vi "Open Protocol.vi"(8 "error in (no error)":errorcluster, 11 "Python Protocol in":refnum<class "Python Protocol.lvclass">) -> (0 "error out":errorcluster, 3 "Python Protocol out":refnum<class "Python Protocol.lvclass">)   [LabVIEW 2012, in "Python Protocol Actor.lvlib" / "Python Protocol.lvclass"]
uses:
  Python Protocol.lvclass
  Python Protocol.lvclass/Python Protocol.ctl
  Read Compiler.vi
  Read Code.vi
  Read Path.vi
  Read Open.vi
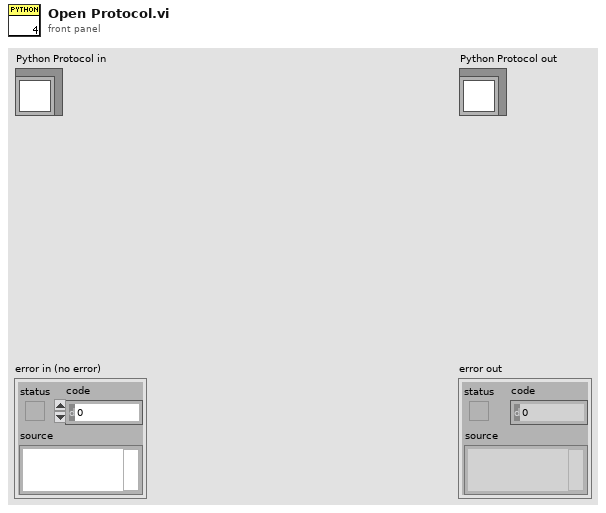
[diagram p1: front panel]
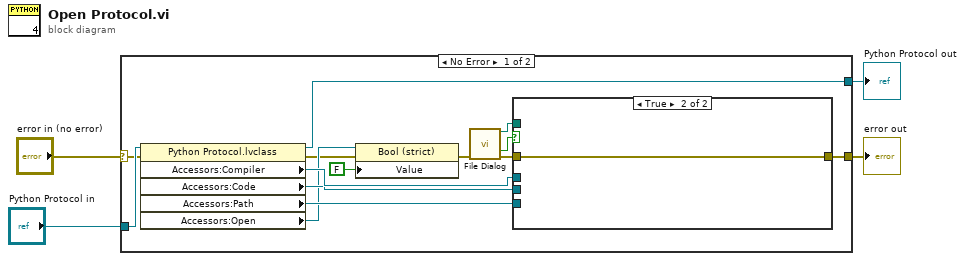
[diagram p0: block diagram]
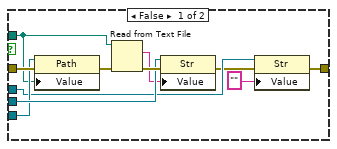
[diagram p2: hidden frame]
diagram:
  n1 = case shown="No Error" "error in (no error)" {
    selector: "error in (no error)" -> [w6 w32]
    tunnel: [w5 w32] -> w3
    tunnel: [w12 w31] -> w1
    tunnel: "Python Protocol in" -> [w13 w31]
    frame No Error {
      n2 = property class="Python Protocol.lvclass"(reference=w13, error in=w6) -> (reference out=w12:refnum<class "Python Protocol.lvclass">, error out=w7:errorcluster, "Accessors:Compiler"=w11:refnum<vi>, "Accessors:Code"=w10:refnum<vi>, "Accessors:Path"=w9:refnum<vi>, "Accessors:Open"=w8:refnum<vi>)
      n3 = property class="Bool (strict)"(reference=w8, error in=w7, "Value"=FALSE) -> (error out=w16:errorcluster)  [unwired: 1 out]
      n4 = call "File Dialog"("error in"=w16) -> ("selected path"=w17:path, "cancelled"=w14:bool, "error out"=w18:errorcluster)  [unwired: 11 in, 1 out]
      n5 = case shown="True" w14 {
        tunnel: w10 -> [w28 _]
        tunnel: w18 -> [w26 w30]
        tunnel: w9 -> [w24 _]
        tunnel: w17 -> [w23 _]
        tunnel: w11 -> [w22 _]
        tunnel: [w20 w30] -> w5
        frame False {
          n6 = property class="Path"(reference=w24, error in=w26, "Value"=w23) -> (error out=w25:errorcluster)  [unwired: 1 out]
          n7 = Read from Text File(file (use dialog)=w23, error in=w25) -> (text=w27:string, error out=w29:errorcluster)  [unwired: 2 in, 2 out]
          n8 = property class="Str"(reference=w28, error in=w29, "Value"=w27) -> (error out=w21:errorcluster)  [unwired: 1 out]
          n9 = property class="Str"(reference=w22, error in=w21, "Value"="") -> (error out=w20:errorcluster)  [unwired: 1 out]
        }
        frame True {
        }
      }
    }
    frame Error {
    }
  }
  "error out" <- w3
  "Python Protocol out" <- w1
